vi "Framework Test.vi"() -> ()   [LabVIEW 2017]
uses:
  Source/DSF Configuration API/1.0.0/Public/Controls/DSF Direction.ctl
  Source/DSF Configuration API/1.0.0/Public/Controls/DSF Timing Info.ctl
  Built/Engine/DSF.Engine.lvlibp/DSF Configuration API/1.0.0/Public/Controls/DSF Settings Info.ctl
  Built/Engine/DSF.Engine.lvlibp/DSF Configuration API/1.0.0/Public/Controls/DSF Data Type.ctl
  <vilib>/Platform/TimedLoop/XDataNode/timing_clust.ctl
  <vilib>/Platform/TimedLoop/XDataNode/nitl_modes.ctl
  <vilib>/Platform/TimedLoop/XDataNode/wakeup.ctl
  Built/Engine/DSF.Engine.lvlibp/Engine/Classes/Debug/DSF.Engine.Debug Flags.FIFO.lvclass
  Built/Engine/DSF.Engine.lvlibp/Engine/Classes/Debug/DSF.Engine.Debug Flags.lvclass
  Built/Engine/DSF.Engine.lvlibp/Engine/Classes/Framework/DSF.Engine.Framework.lvclass
  <vilib>/National Instruments/Memory Manager/Classes/Pointer/Memory.Pointer.lvclass/Memory.Pointer.ctl
  <vilib>/National Instruments/Memory Manager/Classes/Pointer/Memory.Pointer.New.4B.vi
  <vilib>/National Instruments/Memory Manager/Classes/Pointer/Memory.Pointer.Write.0D.U32.vi
  <vilib>/National Instruments/Memory Manager/Classes/Pointer/Memory.Pointer.New.1B.vi
  <vilib>/National Instruments/Memory Manager/Classes/Pointer/Memory.Pointer.Write.0D.Bool.vi
  <vilib>/National Instruments/Memory Manager/Classes/Pointer/Memory.Pointer.Read.0D.I32.vi
  <vilib>/National Instruments/Memory Manager/Classes/Pointer/Memory.Pointer.Read.0D.U32.vi
  <vilib>/National Instruments/Memory Manager/Classes/Pointer/Memory.Pointer.Read.0D.Bool.vi
  <vilib>/National Instruments/Memory Manager/Classes/Pointer/Memory.Pointer.Write.0D.I32.vi
  <vilib>/National Instruments/Memory Manager/Classes/Pointer/Memory.Pointer.Allocate.vi
  <vilib>/National Instruments/Memory Manager/Classes/Pointer/Memory.Pointer.Write.No Check.0D.U32.vi
  <vilib>/National Instruments/Memory Manager/Classes/Pointer/Memory.Pointer.Parameter Check.Null Pointer.vi
  <vilib>/National Instruments/Memory Manager/Classes/Pointer/Memory.Pointer.Parameter Check.Subset.vi
  <vilib>/National Instruments/Memory Manager/Classes/Pointer/Memory.Pointer.Write.No Check.0D.Bool.vi
  <vilib>/National Instruments/Memory Manager/Classes/Pointer/Memory.Pointer.Read.No Check.0D.I32.vi
  <vilib>/National Instruments/Memory Manager/Classes/Pointer/Memory.Pointer.Read.No Check.0D.U32.vi
  <vilib>/National Instruments/Memory Manager/Classes/Pointer/Memory.Pointer.Read.No Check.0D.Bool.vi
  <vilib>/National Instruments/Memory Manager/Classes/Pointer/Memory.Pointer.Write.No Check.0D.I32.vi
  <vilib>/National Instruments/Memory Manager/Classes/Pointer/Memory.Pointer.Set Address.vi
  <vilib>/National Instruments/Memory Manager/Classes/Pointer/Memory.Pointer.Set Size.vi
  <vilib>/National Instruments/Memory Manager/Classes/Pointer/Memory.Pointer.Set Allocated.vi
  <vilib>/National Instruments/Memory Manager/Classes/Pointer/Memory.Pointer.Get Address.vi
  <vilib>/National Instruments/Memory Manager/Classes/Pointer/Memory.Pointer.Errors.vi
  <vilib>/National Instruments/Memory Manager/Classes/Pointer/Memory.Pointer.Errors.Null Pointer.vi
  <vilib>/National Instruments/Memory Manager/Classes/Pointer/Memory.Pointer.Errors.Out of Bounds.vi
  <vilib>/National Instruments/Memory Manager/Classes/Pointer/Memory.Pointer.Get Size.vi
  <vilib>/National Instruments/Memory Manager/Classes/Pointer/Memory.Pointer.Errors.Create Error.vi
  <vilib>/NI/Static Error Handling/VIs/Static Error Handling.Source Buffer.Write.String.vi
  <vilib>/National Instruments/Memory Manager/Classes/Pointer/Memory.Pointer.Errors.Write Pointer Size.vi
  <vilib>/NI/Static Error Handling/VIs/Static Error Handling.Source Buffer.Write.Numeric.Scalar.Base10.vi
  <vilib>/NI/Static Error Handling/VIs/Static Error Handling.Source Buffer.Write.Numeric.Scalar.Base10 (U64).vi
  <vilib>/NI/Static Error Handling/VIs/Static Error Handling.Error Cluster Constant.vi
  <vilib>/NI/Static Error Handling/VIs/Static Error Handling.Error Cluster Constant (512B).vi
  <vilib>/NI/Static Error Handling/VIs/Static Error Handling.Parameters.Status.Set.vi
  <vilib>/NI/Static Error Handling/VIs/Static Error Handling.Parameters.Code.Set.vi
  <vilib>/NI/Static Error Handling/VIs/Static Error Handling.Parameters.VI Source.Set.vi
  <vilib>/National Instruments/Memory Manager/Constants/Memory.Constants.vi
  <vilib>/National Instruments/Memory Manager/Constants/Memory.Constants.Library Name.vi
  <vilib>/National Instruments/Memory Manager/Classes/Pointer/Memory.Pointer.Errors.Get Info.vi
  <vilib>/National Instruments/Memory Manager/Classes/Pointer/Memory.Pointer.lvclass
  <vilib>/platform/TimedLoop/XDataNode/XDataNode.xnode
  <vilib>/Platform/TimedLoop/XDataNode/XDNodeRunTimeDep.lvlib
  Built/Engine/DSF.Engine.lvlibp/Shared/Classes/Framework/DSF.Shared.Configuration.Framework.lvclass
  Built/Engine/DSF.Engine.lvlibp/Engine/Classes/Pointer/DSF.Engine.Pointer.DBL.lvclass
  Built/Engine/DSF.Engine.lvlibp/Engine/Classes/Status/DSF.Engine.Status.Framework.lvclass
  Built/Engine/DSF.Engine.lvlibp/Engine/Classes/Status/DSF.Engine.Status.Framework.Performance.lvclass
  C:/Git/DSF/DSF Core/Built/Engine/DSF.Engine.lvlibp/1abvi3w/vi.lib/National Instruments/Memory Manager/Classes/Pointer/Memory.Pointer.lvclass
  Source/DSF Configuration API/1.0.0/DSF Configuration API.lvlib
  Built/Engine/DSF.Engine.lvlibp/DSF Configuration API/1.0.0/DSF Configuration API.lvlib
panel:
  in  "UDP Rx max size":i32=800
  in  "UDP Rx ports":u16[](array[numeric])=[60000, 60001, 60002, 60003]
  in  "Plugins":T5(array[cluster])=[{"plugin class"="DSF.Transceiver.UDP", "group configs"=[{"direction"=enum."Tx", "timing"={"priority"=100, "decimation"=1, "offset"=0}, "settings"=[], "transfer configs"=[{"random types?"=FALSE, "non-random type"=enum."DBL", "channel count"=100, "settings"=[{"key"="Destination Address", "value"="localhost"}, {"key"="Destination Port", "value"="60000"}]}]}, {"direction"=enum."Tx", "timing"={"priority"=100, "decimation"=2, "offset"=0}, "settings"=[], "transfer configs"=[{"random types?"=FALSE, "non-random type"=enum."DBL", "channel count"=100, "settings"=[{"key"="Destination Address", "value"="localhost"}, {"key"="Destination Port", "value"="60001"}]}]}, {"direction"=enum."Tx", "timing"={"priority"=100, "decimation"=3, "offset"=0}, "settings"=[], "transfer configs"=[{"random types?"=FALSE, "non-random type"=enum."DBL", "channel count"=100, "settings"=[{"key"="Destination Address", "value"="localhost"}, {"key"="Destination Port", "value"="60002"}]}]}, {"direction"=enum."Tx", "timing"={"priority"=100, "decimation"=4, "offset"=0}, "settings"=[], "transfer configs"=[{"random types?"=FALSE, "non-random type"=enum."DBL", "channel count"=100, "settings"=[{"key"="Destination Address", "value"="localhost"}, {"key"="Destination Port", "value"="60003"}]}]}], "plugin timing"={"priority"=100, "decimation"=1, "offset"=0}, "settings"=[{"key"="Local Port", "value"="50000"}]}]
  in  "Infinite Timeouts":bool=TRUE
  out "Framework Error":errorcluster
  out "Tx duration":u32 format="%d us"
  out "Rx duration":u32 format="%d us"
  out "Actual Frequency":dbl format="%.0pHz"
  in  "Transceiver Count":i32=4
  in  "Configuration Path":path=path "C:/Users/Admin/Desktop/test.json"
  out "Framework Iteration":i32 format="%d cycles"
  out "Actual Period":u32 format="%d us"
  in  "Target PCL Period":u32=10000 caption="Target Period" format="%d us"
  in  "stop":bool
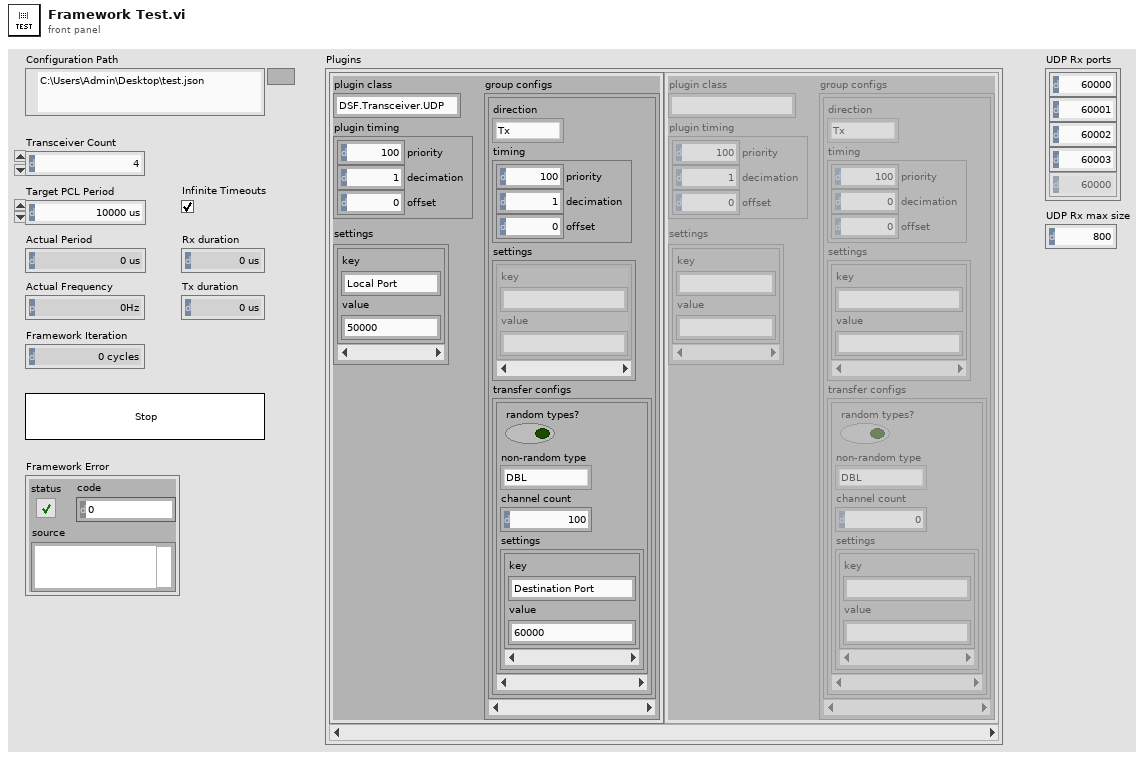
[diagram p1: front panel]
types:
  T1 = typedef "DSF Configuration API.lvlib/DSF Direction.ctl" = enum8{"Tx", "Rx"}
  T2 = typedef "DSF Configuration API.lvlib/DSF Timing Info.ctl" = cluster{"priority":u64, "decimation":u64, "offset":u64}
  T3 = typedef "DSF.Engine.lvlibp/DSF Configuration API.lvlib/DSF Settings Info.ctl" = cluster{"key":string, "value":string}[]
  T4 = typedef "DSF.Engine.lvlibp/DSF Configuration API.lvlib/DSF Data Type.ctl" = enum8{"Bool", "SGL", "DBL", "I8", "I16", "I32", "I64", "U8", "U16", "U32", "U64"}
  T5 = cluster{"plugin class":string, "group configs":cluster{"direction":T1, "timing":T2, "settings":T3, "transfer configs":cluster{"random types?":bool, "non-random type":T4, "channel count":i32, "settings":T3}[]}[], "plugin timing":T2, "settings":T3}[]
  T6 = typedef "DSF.Engine.lvlibp/DSF Configuration API.lvlib/DSF Engine Framework Configuration.ctl" = cluster{"Plugins":T7[]}
  T7 = typedef "DSF.Engine.lvlibp/DSF Configuration API.lvlib/DSF Engine Plugin Configuration.ctl" = cluster{"name":string, "class":string, "cycle timing":T8, "Transfer Groups":T9[], "settings":T3}
  T8 = typedef "DSF.Engine.lvlibp/DSF Configuration API.lvlib/DSF Timing Info.ctl" = cluster{"priority":u64, "decimation":u64, "offset":u64}
  T9 = typedef "DSF.Engine.lvlibp/DSF Configuration API.lvlib/DSF Engine Transfer Group Configuration.ctl" = cluster{"name":string, "direction":T10, "cycle timing":T8, "Transfers":T11[], "settings":T3}
  T10 = typedef "DSF.Engine.lvlibp/DSF Configuration API.lvlib/DSF Direction.ctl" = enum8{"Tx", "Rx"}
  T11 = typedef "DSF.Engine.lvlibp/DSF Configuration API.lvlib/DSF Engine Transfer Configuration.ctl" = cluster{"name":string, "byte order":T12, "channel configurations":T13[], "settings":T3}
  T12 = typedef "DSF.Engine.lvlibp/DSF Configuration API.lvlib/DSF Byte Order.ctl" = enum8{"big-endian", "little-endian"}
  T13 = typedef "DSF.Engine.lvlibp/DSF Configuration API.lvlib/DSF Engine Channel Configuration.ctl" = cluster{"engine offset":u64, "name":string, "data type":T4, "count":u64, "buffer offset":u64, "settings":T3}
  T14 = typedef "XDNodeRunTimeDep.lvlib/timing_clust.ctl" = cluster{"Expected End [f-1]":u64, "Actual End [f-1]":u64, "Finished Late? [f-1]":bool, "Expected End [i-1]":u64, "Actual End [i-1]":u64, "Finished Late? [i-1]":bool, "Expected Start [i]":u64, "Actual Start [i]":u64, "Expected Start [f]":u64, "Actual Start [f]":u64, "Source Name":string, "Structure Name":string, "Period":i64, "Deadline":i64, "Offset":i64, "Start":i64, "Priority":i32, "Timeout":i32, "Mode":T15, "Wakeup Reason":T16, "Error":errorcluster, "Source Type":string, "Secondary Source Type":string, "Global End Time":u64, "Global Start Time":u64, "Frame Duration":u64, "Iteration Duration":u64, "Assigned CPU":i32, "I/O Scan Engine Mode":u32}
  T15 = typedef "XDNodeRunTimeDep.lvlib/nitl_modes.ctl" = enum32{"No Change", "Process missed periods, maintain original phase", "Discard missed periods, maintain original phase", "Process missed periods, ignore original phase", "Discard missed periods, ignore original phase"}
  T16 = typedef "XDNodeRunTimeDep.lvlib/wakeup.ctl" = enum32{"Normal", "Aborted", "Asynchronous wakeup", "Timing source error", "Timed loop error", "Timeout"}
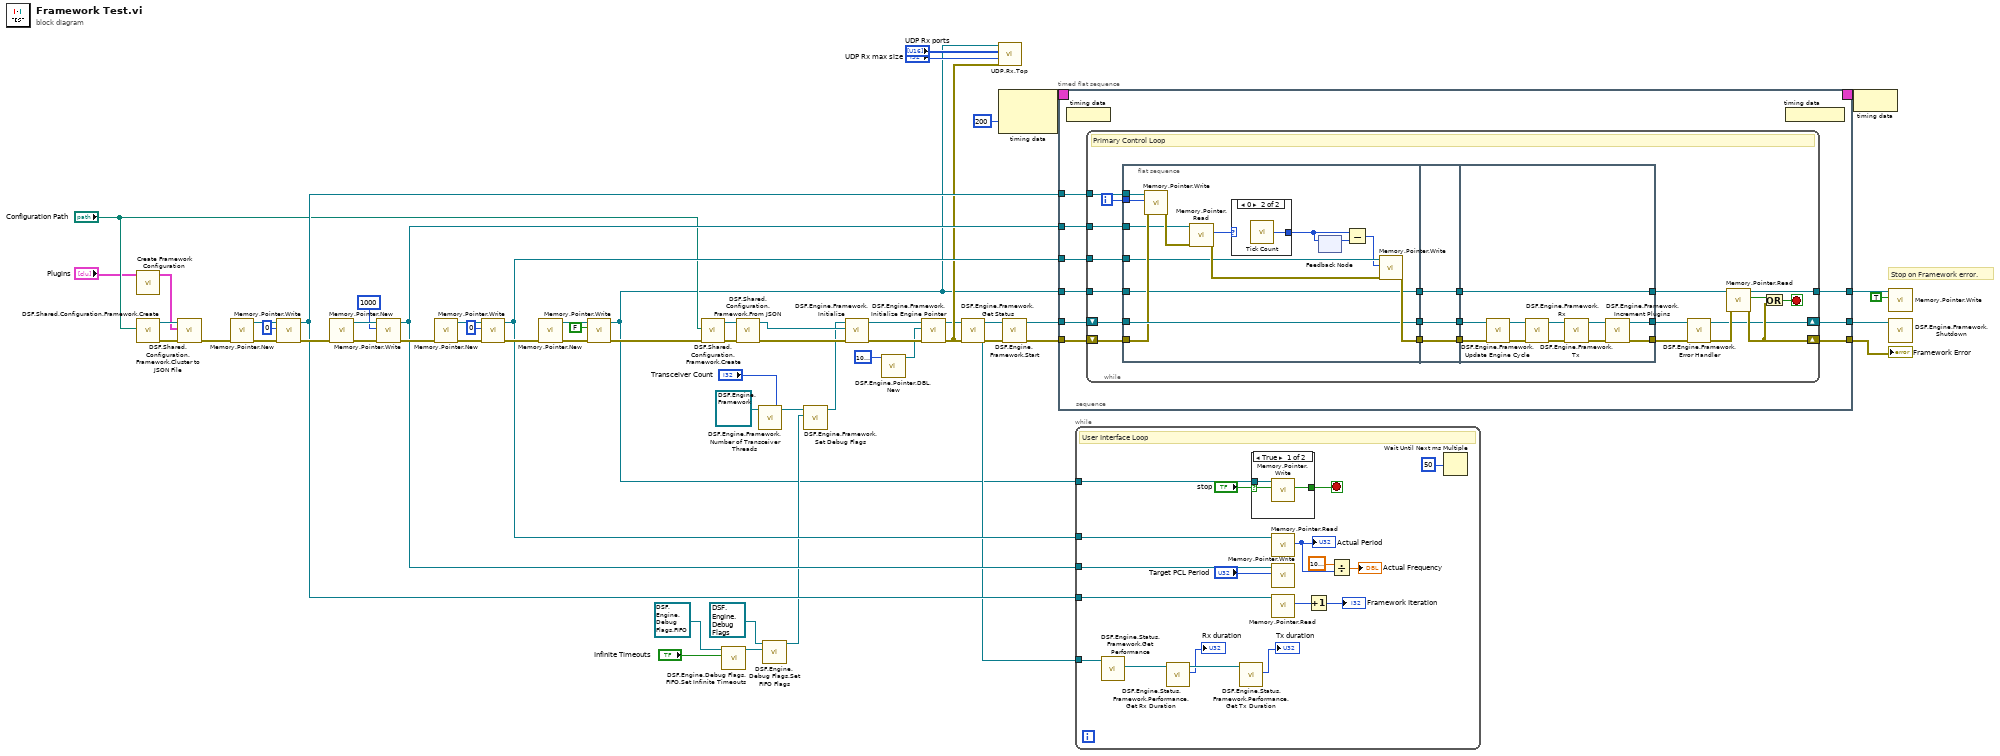
[diagram p0: block diagram]
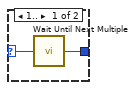
[diagram p2: hidden frame]
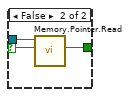
[diagram p3: hidden frame]
diagram:
  # "Stop on Framework error."
  n1 = call "Create Framework Configuration.vi"("Plugins"="Plugins") -> ("Framework Configuration"=w8:T6)  [unwired: 10 in]
  n2 = call "DSF.Shared.Configuration.Framework.Create.vi"("configuration path"="Configuration Path") -> ("error out"=w32:errorcluster, "Framework Configuration"=w33:refnum<class "DSF.Shared.Configuration.Framework.lvclass">)  [unwired: 9 in]
  n3 = call "DSF.Shared.Configuration.Framework.Cluster to JSON File.vi"("error in (no error)"=w32, "Framework Configuration"=w8, "Framework Configuration in"=w33) -> ("error out"=w31:errorcluster)  [unwired: 7 in, 1 out]
  n4 = call-poly <vilib>:"Memory.Pointer.New.vi"("error in (no error)"=w31) -> ("error out"=w39:errorcluster, "Pointer"=w40:refnum<class "Memory.Pointer.lvclass">)  [unwired: 9 in]
  n5 = call-poly <vilib>:"Memory.Pointer.Write.vi"("error in (no error)"=w39, "value"=u32 0, "Pointer in"=w40) -> ("error out"=w38:errorcluster, "Pointer out"=w35:refnum<class "Memory.Pointer.lvclass">)  [unwired: 5 in, 2 out]
  n6 = call-poly <vilib>:"Memory.Pointer.New.vi"("error in (no error)"=w38) -> ("error out"=w46:errorcluster, "Pointer"=w47:refnum<class "Memory.Pointer.lvclass">)  [unwired: 9 in]
  n7 = call-poly <vilib>:"Memory.Pointer.Write.vi"("error in (no error)"=w46, "value"=u32 1000, "Pointer in"=w47) -> ("error out"=w45:errorcluster, "Pointer out"=w41:refnum<class "Memory.Pointer.lvclass">)  [unwired: 5 in, 2 out]
  n8 = call-poly <vilib>:"Memory.Pointer.New.vi"("error in (no error)"=w45) -> ("error out"=w44:errorcluster, "Pointer"=w48:refnum<class "Memory.Pointer.lvclass">)  [unwired: 9 in]
  n9 = call-poly <vilib>:"Memory.Pointer.Write.vi"("error in (no error)"=w44, "value"=u32 0, "Pointer in"=w48) -> ("error out"=w43:errorcluster, "Pointer out"=w42:refnum<class "Memory.Pointer.lvclass">)  [unwired: 5 in, 2 out]
  n10 = call-poly <vilib>:"Memory.Pointer.New.vi"("error in (no error)"=w43) -> ("error out"=w51:errorcluster, "Pointer"=w50:refnum<class "Memory.Pointer.lvclass">)  [unwired: 9 in]
  n11 = call-poly <vilib>:"Memory.Pointer.Write.vi"("error in (no error)"=w51, "value"=FALSE, "Pointer in"=w50) -> ("error out"=w34:errorcluster, "Pointer out"=w3:refnum<class "Memory.Pointer.lvclass">)  [unwired: 5 in, 2 out]
  n12 = call "DSF.Shared.Configuration.Framework.Create.vi"("error in (no error)"=w34, "configuration path"="Configuration Path") -> ("error out"=w36:errorcluster, "Framework Configuration"=w37:refnum<class "DSF.Shared.Configuration.Framework.lvclass">)  [unwired: 8 in]
  n13 = call "DSF.Engine.Debug Flags.FIFO.Set Infinite Timeouts.vi"("infinite timeouts"="Infinite Timeouts", "FIFO Debug Flags in"=refnum<class "DSF.Engine.Debug Flags.FIFO.lvclass"> refnum) -> ("FIFO Debug Flags out"=w26:refnum<class "DSF.Engine.Debug Flags.FIFO.lvclass">)  [unwired: 9 in]
  n14 = call "DSF.Shared.Configuration.Framework.From JSON.vi"("error in (no error)"=w36, "Framework Configuration in"=w37) -> ("error out"=w58:errorcluster, "Framework Configuration out"=w21:refnum<class "DSF.Shared.Configuration.Framework.lvclass">)  [unwired: 8 in]
  n15 = call "DSF.Engine.Framework.Number of Transceiver Threads.vi"("transceiver count"="Transceiver Count", "Framework in"=refnum<class "DSF.Engine.Framework.lvclass"> refnum) -> ("Framework out"=w27:refnum<class "DSF.Engine.Framework.lvclass">)  [unwired: 8 in, 1 out]
  n16 = call "DSF.Engine.Debug Flags.Set FIFO Flags.vi"("FIFO"=w26, "Debug Flags in"=refnum<class "DSF.Engine.Debug Flags.lvclass"> refnum) -> ("Debug Flags out"=w22:refnum<class "DSF.Engine.Debug Flags.lvclass">)  [unwired: 9 in]
  n17 = call "DSF.Engine.Framework.Set Debug Flags.vi"("Debug Flags"=w22, "Framework in"=w27) -> ("Framework out"=w12:refnum<class "DSF.Engine.Framework.lvclass">)  [unwired: 9 in]
  n18 = call "DSF.Engine.Framework.Initialize.vi"("error in (no error)"=w58, "Framework Configuration"=w21, "Framework type"=w12) -> ("error out"=w14:errorcluster, "Framework out"=w15:refnum<class "DSF.Engine.Framework.lvclass">)  [unwired: 7 in]
  n19 = call "DSF.Engine.Pointer.DBL.New.vi"("channel count"=u64 1000000) -> ("DBL Pointer out"=w11:refnum<class "DSF.Engine.Pointer.DBL.lvclass">)  [unwired: 9 in, 1 out]
  n20 = call "DSF.Engine.Framework.Initialize Engine Pointer.vi"("error in (no error)"=w14, "Engine Pointer"=w11, "Framework in"=w15) -> ("error out"=w7:errorcluster, "Framework out"=w6:refnum<class "DSF.Engine.Framework.lvclass">)  [unwired: 7 in]
  n21 = call "DSF.Engine.Framework.Get Status.vi"("Framework in"=w6) -> ("Status"=w10:refnum<class "DSF.Engine.Status.Framework.lvclass">, "Framework out"=w13:refnum<class "DSF.Engine.Framework.lvclass">)  [unwired: 9 in]
  n22 = call "UDP.Rx.Top.vi"("error in (no error)"=w7, "max size (800)"="UDP Rx max size", "ports"="UDP Rx ports", "Stop Pointer"=w3) -> ()  [unwired: 7 in, 1 out]
  n23 = node-c288(200 ("Priority")) -> (w53:T14)  [unwired: 1 in]
  n24 = call "DSF.Engine.Framework.Start.vi"("error in (no error)"=w7, "Framework in"=w13) -> ("error out"=w56:errorcluster, "Framework out"=w57:refnum<class "DSF.Engine.Framework.lvclass">)  [unwired: 8 in]
  n25 = timed-sequence {
    timing: w53 -> [_]
    timing-out: [_] -> w52
    tunnel: w57 -> [w67]
    tunnel: w56 -> [w66]
    tunnel: [w65] -> w55
    tunnel: [w64] -> w54
    tunnel: w3 -> [w63]
    tunnel: w41 -> [w62]
    tunnel: w42 -> [w61]
    tunnel: w35 -> [w60]
    tunnel: [w59] -> w2
    n26 = timed-flat-sequence {
      tunnel: w67 -> [w76]
      tunnel: w66 -> [w75]
      tunnel: [w74] -> w65
      tunnel: [w73] -> w64
      tunnel: w63 -> [w72]
      tunnel: w62 -> [w71]
      tunnel: w61 -> [w70]
      tunnel: w60 -> [w69]
      tunnel: [w68] -> w59
      n27 = node-c288() -> ()  [unwired: 1 in]
      n28 = while {
        shift-right: [w77] -> w74
        shift-left: w76 -> [w97]
        shift-right: [w91] -> w73
        shift-left: w75 -> [w98]
        tunnel: w72 -> [w96]
        tunnel: w71 -> [w94]
        tunnel: w70 -> [w93]
        tunnel: w69 -> [w89]
        tunnel: [w81] -> w68
        i -> [w88]
        stop <- w90 stop-if-true
        # "Primary Control Loop"
        n29 = flat-sequence {
          tunnel: w98 -> [w107]
          tunnel: w97 -> [w110]
          tunnel: w96 -> [w103]
          tunnel: [w111] -> w87
          tunnel: [w110] -> w85
          tunnel: [w103] -> w83
          tunnel: w94 -> [w105]
          tunnel: w93 -> [w104]
          tunnel: w89 -> [w108]
          tunnel: w88 -> [w101]
          tunnel: w87 -> [w118]
          tunnel: [w118] -> w86
          tunnel: w85 -> [w117]
          tunnel: [w117] -> w84
          tunnel: w83 -> [w116]
          tunnel: [w116] -> w82
          tunnel: w86 -> [w121]
          tunnel: w84 -> [w122]
          tunnel: w82 -> [w123]
          tunnel: [w123] -> w95
          tunnel: [w125] -> w80
          tunnel: [w124] -> w79
          frame #0 {
            n30 = call-poly <vilib>:"Memory.Pointer.Write.vi"("error in (no error)"=w107, "value"=w101, "Pointer in"=w108) -> ("error out"=w106:errorcluster)  [unwired: 5 in, 3 out]
            n31 = call-poly <vilib>:"Memory.Pointer.Read.vi"("error in (no error)"=w106, "Pointer in"=w105) -> ("error out"=w109:errorcluster, "value out"=w99:u32)  [unwired: 6 in, 2 out]
            n32 = case shown="0" w99 {
              selector: w99 -> [w113 _]
              tunnel: [w114 w115] -> w102
              frame 1.. {
                n33 = call "Wait Until Next Multiple"("Count(uSec)"=w113) -> ("Tick Count(uSec)"=w114:u32)
              }
              frame 0 {
                n34 = call "Tick Count"() -> ("Tick Count(uSec)"=w115:u32)
              }
            }
            n35 = feedback #1() -> (w112:u32)  [unwired: 1 in]
            n36 = feedback-in #1(w102) -> ()
            n37 = Subtract(x=w102, y=w112) -> (x-y=w100:u32)
            n38 = call-poly <vilib>:"Memory.Pointer.Write.vi"("error in (no error)"=w109, "value"=w100, "Pointer in"=w104) -> ("error out"=w111:errorcluster)  [unwired: 5 in, 3 out]
          }
          frame #1 {
          }
          frame #2 {
            n39 = call-dynamic "DSF.Engine.Framework.Update Engine Cycle.vi"("error in (no error)"=w121, "Framework in"=w122) -> ("error out"=w119:errorcluster, "Framework out"=w120:refnum<class "DSF.Engine.Framework.lvclass">)  [unwired: 8 in]
            n40 = call "DSF.Engine.Framework.Rx.vi"("error in (no error)"=w119, "Framework in"=w120) -> ("error out"=w129:errorcluster, "Framework out"=w128:refnum<class "DSF.Engine.Framework.lvclass">)  [unwired: 8 in]
            n41 = call "DSF.Engine.Framework.Tx.vi"("error in (no error)"=w129, "Framework in"=w128) -> ("error out"=w126:errorcluster, "Framework out"=w127:refnum<class "DSF.Engine.Framework.lvclass">)  [unwired: 8 in]
            n42 = call "DSF.Engine.Framework.Increment Plugins.vi"("error in (no error)"=w126, "Framework in"=w127) -> ("error out"=w124:errorcluster, "Framework out"=w125:refnum<class "DSF.Engine.Framework.lvclass">)  [unwired: 8 in]
          }
        }
        n43 = call "DSF.Engine.Framework.Error Handler.vi"("error in (no error)"=w79, "Framework in"=w80) -> ("error out"=w78:errorcluster, "Framework out"=w77:refnum<class "DSF.Engine.Framework.lvclass">)  [unwired: 8 in]
        n44 = call-poly <vilib>:"Memory.Pointer.Read.vi"("error in (no error)"=w78, "Pointer in"=w95) -> ("error out"=w91:errorcluster, "value out"=w92:bool, "Pointer out"=w81:refnum<class "Memory.Pointer.lvclass">)  [unwired: 6 in, 1 out]
        n45 = Or(x=w92, y=w91) -> (x .or. y?=w90:bool)
      }
      n46 = node-c288() -> ()  [unwired: 1 out]
    }
  }
  "Framework Error" <- w54
  n47 = while {
    tunnel: w3 -> [w148]
    tunnel: w42 -> [w145]
    tunnel: w41 -> [w146]
    tunnel: w35 -> [w142]
    tunnel: w10 -> [w140]
    stop <- w149 stop-if-true
    # "User Interface Loop"
    n48 = call "DSF.Engine.Status.Framework.Get Performance.vi"("Framework Status in"=w140) -> ("Framework Performance"=w139:refnum<class "DSF.Engine.Status.Framework.Performance.lvclass">)  [unwired: 9 in, 1 out]
    n49 = call "DSF.Engine.Status.Framework.Performance.Get Rx Duration.vi"("Framework Performance in"=w139) -> ("rx duration"=→"Rx duration":u32, "Framework Performance out"=w138:refnum<class "DSF.Engine.Status.Framework.Performance.lvclass">)  [unwired: 8 in, 1 out]
    n50 = call "DSF.Engine.Status.Framework.Performance.Get Tx Duration.vi"("Framework Performance in"=w138) -> ("tx duration"=→"Tx duration":u32)  [unwired: 8 in, 2 out]
    n51 = case shown="True" "stop" {
      selector: "stop" -> [w150 w153]
      tunnel: [w152 w155] -> w149
      tunnel: w148 -> [w151 w154]
      frame True {
        n52 = call-poly <vilib>:"Memory.Pointer.Write.vi"("value"=w150, "Pointer in"=w151) -> ("value"=w152:bool)  [unwired: 6 in, 3 out]
      }
      frame False {
        n53 = call-poly <vilib>:"Memory.Pointer.Read.vi"("value in"=w153, "Pointer in"=w154) -> ("value out"=w155:bool)  [unwired: 6 in, 3 out]
      }
    }
    n54 = call-poly <vilib>:"Memory.Pointer.Read.vi"("Pointer in"=w145) -> ("value out"=w135:u32)  [unwired: 7 in, 3 out]
    "Actual Period" <- w135
    n55 = call-poly <vilib>:"Memory.Pointer.Write.vi"("value"="Target PCL Period", "Pointer in"=w146) -> ()  [unwired: 6 in, 4 out]
    n56 = call-poly <vilib>:"Memory.Pointer.Read.vi"("Pointer in"=w142) -> ("value out"=w134:i32)  [unwired: 7 in, 3 out]
    n57 = Increment(x=w134) -> (x+1=→"Framework Iteration":i32)
    n58 = Divide(x=1000000.0, y=w135) -> (x/y=→"Actual Frequency":dbl)
    n59 = Wait Until Next ms Multiple(millisecond multiple=u32 50 ("milliseconds to wait")) -> ()  [unwired: 1 out]
  }
  n60 = node-c288(w52) -> ()
  n61 = call-poly <vilib>:"Memory.Pointer.Write.vi"("value"=TRUE, "Pointer in"=w2) -> ()  [unwired: 6 in, 4 out]
  n62 = call "DSF.Engine.Framework.Shutdown.vi"("Framework in"=w55) -> ()  [unwired: 9 in, 2 out]
